vi "Set Current Directory To Library Folder.vi"(8 "error in (no error)":errorcluster) -> (0 "error out":errorcluster)   [LabVIEW 2020]
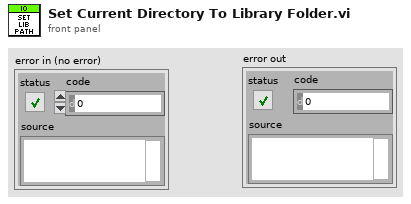
[diagram p1: front panel]
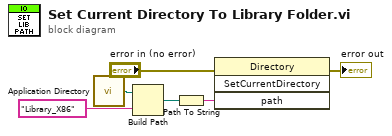
[diagram p0: block diagram]
diagram:
  n1 = call <vilib>:"Application Directory.vi"() -> ("Application Directory"=w6:path)
  n2 = Build Path(base path=w6, name or relative path="Library_X86") -> (appended path=w4:path)
  n3 = Path To String(path=w4) -> (string=w3:string)
  n4 = invoke class="Directory" method="SetCurrentDirectory"(error in="error in (no error)", "path"=w3) -> (error out=→"error out":errorcluster)  [unwired: 2 in, 3 out]
